vi "CrawlingState.vi"(8 "error in (no error)":errorcluster, 9 "Cluster in":T2, 10 "Enum in":T1, 11 "Actual Start [i]":i64) -> (0 "error out":errorcluster, 2 "Cluster out":T2, 3 "Enum":T1)   [LabVIEW 2018]
uses:
  Type_Def/Type_Def Actuator Controls.ctl
  Type_Def/Type_Def ControlState.ctl
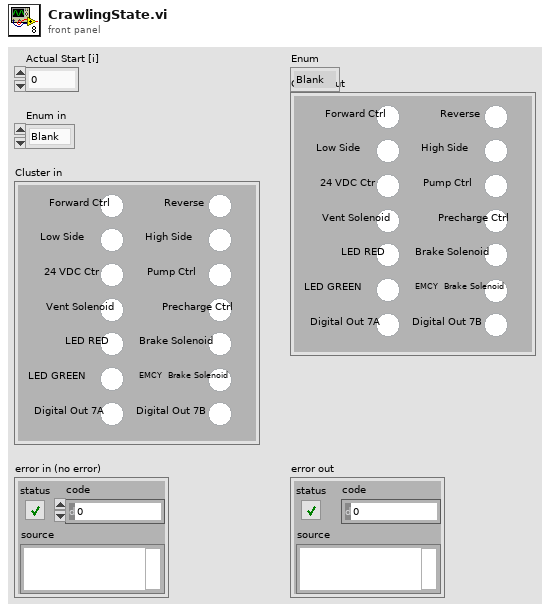
[diagram p1: front panel]
types:
  T1 = typedef "Type_Def ControlState.ctl" = enum16{"Blank", "Systems Check", "Idle", "Ready", "Pushing", "CrawlingPrecharge", "Braking", "Fault", "Boot Up", "Crawling", "Shutdown", "Service Push", "Service Wait", "Vent", "Precharge"}
  T2 = typedef "Type_Def Actuator Controls.ctl" = cluster{"Reverse ":bool, "Precharge Ctrl":bool, "Pump Ctrl":bool, "24 VDC Ctr":bool, "Vent Solenoid":bool, "Brake Solenoid":bool, "EMCY  Brake Solenoid":bool, "Digital Out 7B ":bool, "Forward Ctrl":bool, " Low Side":bool, "High Side":bool, "LED RED":bool, "LED GREEN":bool, " Digital Out 7A":bool}
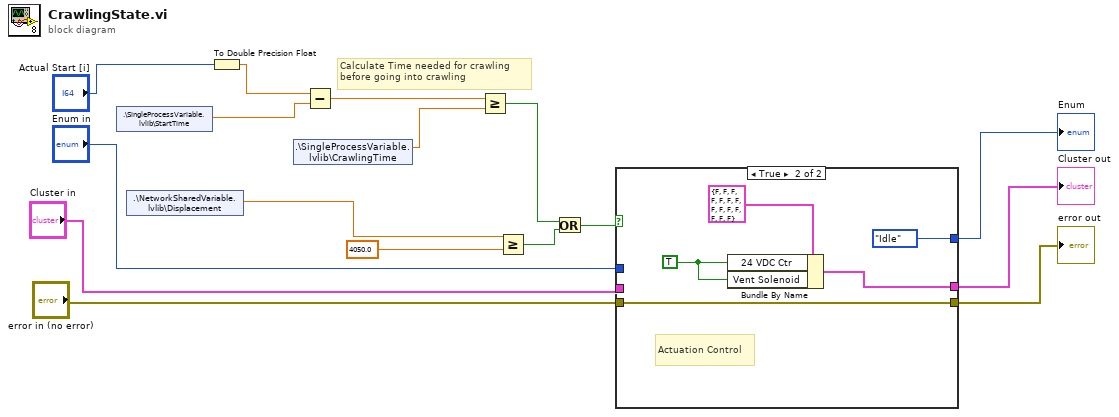
[diagram p0: block diagram]
diagram:
  # "Calculate Time needed for crawling \nbefore going into crawling"
  n1 = shared-variable ".\\SingleProcessVariable.lvlib\\StartTime"() -> (w9:dbl)  [unwired: 1 in, 1 out]
  n2 = shared-variable ".\\NetworkSharedVariable.lvlib\\Displacement"() -> (w15:dbl)  [unwired: 1 in, 1 out]
  n3 = To Double Precision Float(number="Actual Start [i]") -> (double precision float=w1:dbl)
  n4 = shared-variable ".\\SingleProcessVariable.lvlib\\CrawlingTime"() -> (w16:dbl)  [unwired: 1 in, 1 out]
  n5 = Subtract(x=w1, y=w9) -> (x-y=w10:dbl)
  n6 = Greater Or Equal?(x=w10, y=w16) -> (x >= y?=w11:bool)
  n7 = Greater Or Equal?(x=w15, y=4050.0) -> (x >= y?=w13:bool)
  n8 = Or(x=w11, y=w13) -> (x .or. y?=w14:bool)
  n9 = case shown="True" w14 {
    tunnel: "Enum in" -> [w19 _]
    tunnel: [w19 Type_Def_ControlState."Idle"] -> w4
    tunnel: "Cluster in" -> [w18 _]
    tunnel: [w18 w23] -> w6
    tunnel: [w17 w22] -> w7
    tunnel: "error in (no error)" -> [w17 w22]
    frame False {
    }
    frame True {
      w21 = TRUE ("Brake Valve")
      # "Actuation Control"
      n10 = Bundle By Name(cluster=T2 {"Reverse "=FALSE, "Precharge Ctrl"=FALSE, "Pump Ctrl"=FALSE, "24 VDC Ctr"=FALSE, "Vent Solenoid"=FALSE, "Brake Solenoid"=FALSE, "EMCY  Brake Solenoid"=FALSE, "Digital Out 7B "=FALSE, "Forward Ctrl"=FALSE, " Low Side"=FALSE, "High Side"=FALSE, "LED RED"=FALSE, "LED GREEN"=FALSE, " Digital Out 7A"=FALSE} ("Cluster in 2"), "24 VDC Ctr"=w21, "Vent Solenoid"=w21) -> (w23:T2)
    }
  }
  "error out" <- w7
  "Cluster out" <- w6
  "Enum" <- w4
